vi "Running_as_top_level.vi"(0 "Vi path name":path) -> (1 "Top Level":bool, 2 "Execution:State":T1(ring))   [LabVIEW 2015]
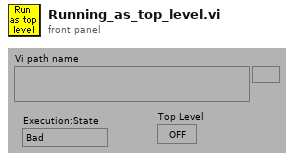
[diagram p1: front panel]
types:
  T1 = enum32{"Bad", "Idle", "Run top level", "Running"}
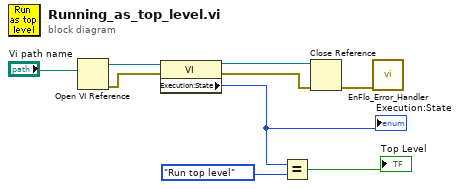
[diagram p0: block diagram]
diagram:
  n1 = Open VI Reference(vi path="Vi path name") -> (vi reference=w9:refnum<vi>, error out=w8:errorcluster)  [unwired: 1 in, 4 out]
  n2 = property class="VI"(reference=w9, error in=w8) -> (reference out=w7:refnum<vi>, error out=w6:errorcluster, "Execution:State"=w3:T1)
  "Execution:State" <- w3
  n3 = Equal?(x=w3, y=T1."Run top level" ("Exec.State")) -> (x = y?=→"Top Level":bool)
  n4 = Close Reference(reference=w7, error in (no error)=w6) -> (error out=w4:errorcluster)
  n5 = call "EnFlo_Error_Handler.vi"("error in (no error)"=w4) -> ()  [unwired: 2 in, 3 out]
